vi "Post Temperature UIMessage.vi"(8 "error in (no error)":errorcluster, 10 "Temperature":dbl, 11 "SequenceContext in":refnum<k7>) -> (0 "error out":errorcluster, 3 "SequenceContext out":refnum<k7>)   [LabVIEW 2013]
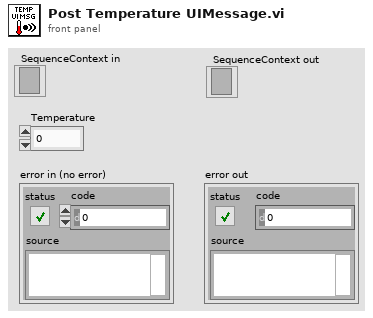
[diagram p1: front panel]
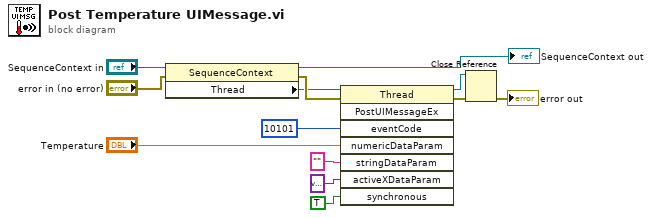
[diagram p0: block diagram]
diagram:
  n1 = property class="SequenceContext"(reference="SequenceContext in", error in="error in (no error)") -> (reference out=→"SequenceContext out":refnum<k7>, error out=w10:errorcluster, "Thread"=w3:refnum<k7>)
  n2 = invoke class="Thread" method="PostUIMessageEx"(reference=w3, error in=w10, "eventCode"=10101 ("DMM Channel"), "numericDataParam"="Temperature", "stringDataParam"="", "activeXDataParam"=variant, "synchronous"=TRUE) -> (reference out=w13:refnum<k7>, error out=w11:errorcluster)  [unwired: 1 in, 6 out]
  n3 = Close Reference(reference=w13, error in (no error)=w11) -> (error out=→"error out":errorcluster)
